vi "return actor number.vi"(11 "Template in":refnum<class "Template.lvclass">) -> (3 "Actor number":u32)   [LabVIEW 2020, in "Template.lvlib" / "Template.lvclass"]
doc: "Returns this actor number to filter for configuration steps"
uses:
  Template.lvclass
  Template.lvclass/Template.ctl
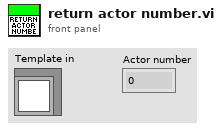
[diagram p1: front panel]
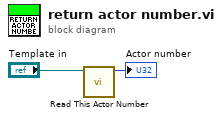
[diagram p0: block diagram]
diagram:
  n1 = call "Read This Actor Number.vi"("Template in"="Template in") -> ("This Actor Number"=→"Actor number":u32)  [unwired: 10 in]
